vi "Print Error.vi"(4 "Filter -2206? (T)":bool=TRUE, 6 "Custom Device? (T)":bool=TRUE, 8 "error out":errorcluster, 10 "Note (empty)":string, 11 "Your code's public name":string) -> ()   [LabVIEW 2023, in "Ethernet IP Custom Device Custom Device.lvlib"]
doc: "Prints error information out to the console. Provide your code's public name. For example, if your code is about J1939, put that here so the user knows what this printed error information has to do with.\n\nIf this is not a NI VeriStand custom device, write false to the Custom Device? input. This will change the error output.\n\nIf the 'note' field is empty, it is not printed to the console.\n\nExample output 1:\n******J1939 ERROR******\nSource: blah.vi\nCode: 535\n******J1939 ERROR******\n\nExample output 2:\n******XCP and CCP Master CUSTOM DEVICE ERROR******\nSource: blah.vi\nCode: 535\nUser Note: before write\n******XCP and CCP Master CUSTOM DEVICE ERROR******"
uses:
  Ethernet IP Custom Device Custom Device.lvlib
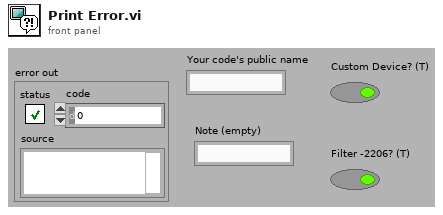
[diagram p1: front panel]
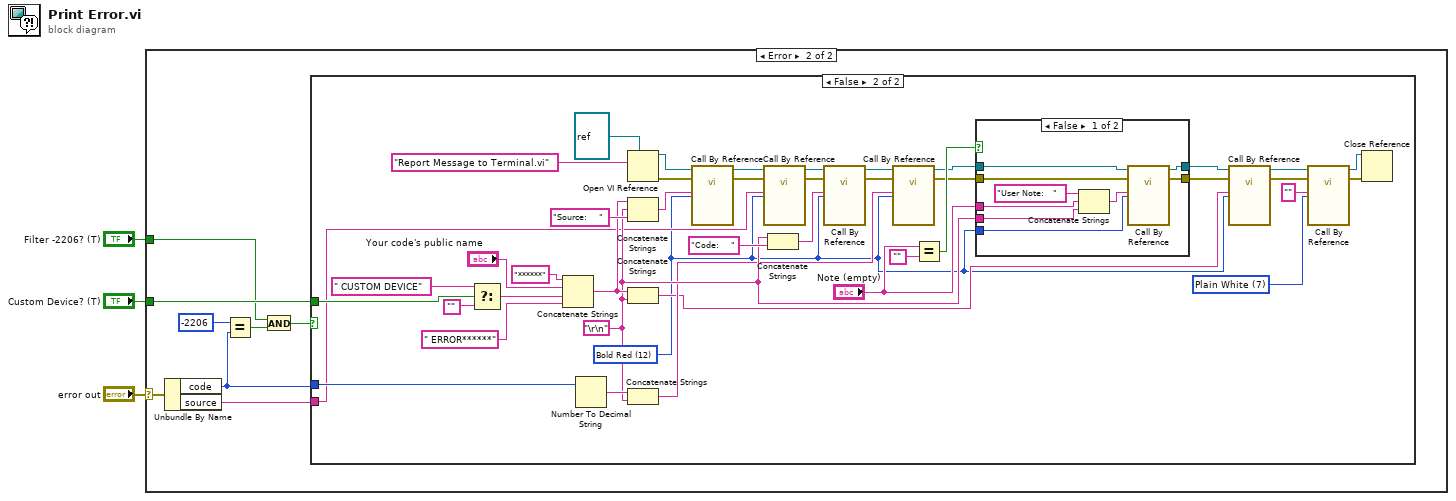
[diagram p0: block diagram]
diagram:
  n1 = case shown="Error" "error out" {
    selector: "error out" -> [_ w11]
    tunnel: "Custom Device? (T)" -> [_ w10]
    tunnel: "Filter -2206? (T)" -> [_ w5]
    frame No Error {
    }
    frame Error {
      n2 = Unbundle By Name(w11) -> ("code"=w8:i32, "source"=w9:string)
      n3 = Equal?(x=-2206, y=w8) -> (x = y?=w6:bool)
      n4 = And(x=w5, y=w6) -> (x .and. y?=w4:bool)
      n5 = case shown="False" w4 {
        tunnel: w8 -> [_ w53]
        tunnel: w10 -> [_ w38]
        tunnel: w9 -> [_ w30]
        frame True {
        }
        frame False {
          w33 = u16 7 items=["Plain White"=7, "Bold White"=15, "Bold Blue"=9, "Bold Green"=10, "Bold Red"=12] ("Color (Plain White)")
          w13 = u16 12 items=["Plain White"=7, "Bold White"=15, "Bold Blue"=9, "Bold Green"=10, "Bold Red"=12] ("Color (Plain White)")
          w41 = "\r\n"
          n6 = Select(t=" CUSTOM DEVICE" ("String"), s=w38, f="") -> (s? t:f=w39:string)
          n7 = Concatenate Strings("******" ("String"), "Your code's public name", w39, " ERROR******" ("String")) -> (w45:string)
          n8 = Number To Decimal String(number=w53) -> (decimal integer string=w50:string)  [unwired: 1 in]
          n9 = Open VI Reference(type specifier VI Refnum (for type only)=refnum<vi> refnum, vi path="Report Message to Terminal.vi") -> (vi reference=w28:refnum<vi>, error out=w27:errorcluster)  [unwired: 1 in, 3 out]
          n10 = Concatenate Strings(w45, w41, "Source:    " ("String")) -> (w32:string)
          n11 = Concatenate Strings(w45, w41) -> (w14:string)
          n12 = Concatenate Strings(w50, w41) -> (w23:string)
          n13 = call-by-ref "?"(reference=w28, error in=w27, "Color (Plain White)"=w13, "Message"=w32) -> (reference out=w29:refnum<vi>, error out=w31:errorcluster)  [unwired: 9 in, 1 out]
          n14 = call-by-ref "?"(reference=w29, error in=w31, "Color (Plain White)"=w13, "Message"=w30) -> (reference out=w24:refnum<vi>, error out=w25:errorcluster)  [unwired: 9 in, 1 out]
          n15 = Concatenate Strings(w41, "Code:    " ("String")) -> (w26:string)
          n16 = call-by-ref "?"(reference=w24, error in=w25, "Color (Plain White)"=w13, "Message"=w26) -> (reference out=w22:refnum<vi>, error out=w21:errorcluster)  [unwired: 9 in, 1 out]
          n17 = call-by-ref "?"(reference=w22, error in=w21, "Color (Plain White)"=w13, "Message"=w23) -> (reference out=w19:refnum<vi>, error out=w20:errorcluster)  [unwired: 9 in, 1 out]
          n18 = Equal?(x="Note (empty)", y="") -> (x = y?=w43:bool)
          n19 = case shown="False" w43 {
            tunnel: "Note (empty)" -> [w61 _]
            tunnel: w41 -> [w60 _]
            tunnel: [w57 w64] -> w18
            tunnel: w20 -> [w59 w64]
            tunnel: w19 -> [w56 w63]
            tunnel: [w55 w63] -> w15
            tunnel: w13 -> [w54 _]
            frame False {
              n20 = Concatenate Strings("User Note:   " ("string"), w61, w60) -> (w58:string)
              n21 = call-by-ref "?"(reference=w56, error in=w59, "Color (Plain White)"=w54, "Message"=w58) -> (reference out=w55:refnum<vi>, error out=w57:errorcluster)  [unwired: 9 in, 1 out]
            }
            frame True {
            }
          }
          n22 = call-by-ref "?"(reference=w15, error in=w18, "Color (Plain White)"=w13, "Message"=w14) -> (reference out=w16:refnum<vi>, error out=w17:errorcluster)  [unwired: 9 in, 1 out]
          n23 = call-by-ref "?"(reference=w16, error in=w17, "Color (Plain White)"=w33, "Message"="") -> (reference out=w34:refnum<vi>, error out=w35:errorcluster)  [unwired: 9 in, 1 out]
          n24 = Close Reference(reference=w34, error in (no error)=w35) -> ()  [unwired: 1 out]
        }
      }
    }
  }
